vi "TestPrinter.vi"() -> ()   [LabVIEW 2020]
panel:
  in  "ID":string="0"
  in  "SN":string="FFF"
  in  "Print":string
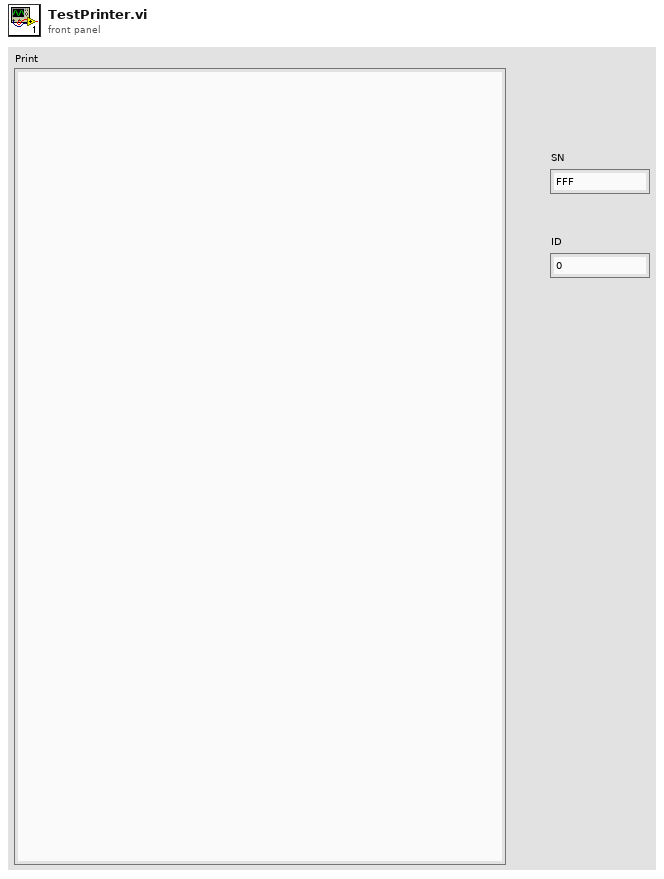
[diagram p1: front panel]
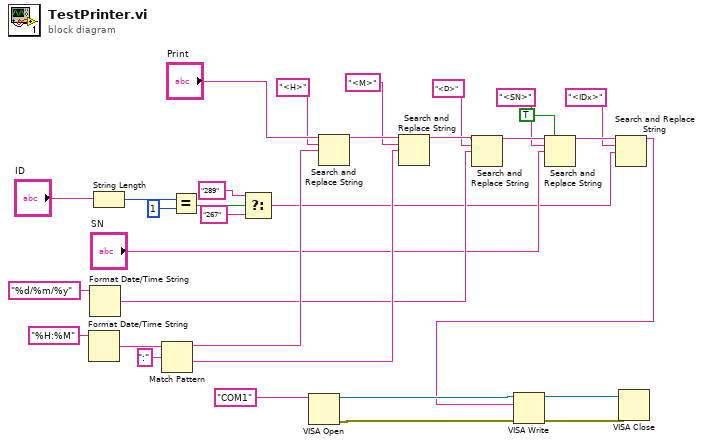
[diagram p0: block diagram]
diagram:
  n1 = Format Date/Time String(time format string (%c)="%H:%M") -> (date/time string=w28:string)  [unwired: 2 in]
  n2 = Format Date/Time String(time format string (%c)="%d/%m/%y") -> (date/time string=w17:string)  [unwired: 2 in]
  n3 = String Length(string="ID") -> (length=w9:i32)
  n4 = Match Pattern(string=w28, regular expression=":") -> (before substring=w22:string, after substring=w19:string)  [unwired: 1 in, 2 out]
  n5 = Equal?(x=w9, y=1) -> (x = y?=w4:bool)
  n6 = Select(t="289", s=w4, f="267") -> (s? t:f=w1:string)
  n7 = VISA Open(VISA resource name="COM1") -> (VISA resource name=w30:refnum<visa-resource-name>, error out=w31:errorcluster)  [unwired: 4 in]
  n8 = Search and Replace String(input string="Print", search string="<H>", replace string=w22) -> (result string=w21:string)  [unwired: 5 in, 3 out]
  n9 = Search and Replace String(input string=w21, search string="<M>", replace string=w19) -> (result string=w16:string)  [unwired: 5 in, 3 out]
  n10 = Search and Replace String(input string=w16, search string="<D>", replace string=w17) -> (result string=w14:string)  [unwired: 5 in, 3 out]
  n11 = Search and Replace String(replace all?=TRUE ("replace all? (F)"), input string=w14, search string="<SN>", replace string="SN") -> (result string=w7:string)  [unwired: 4 in, 3 out]
  n12 = Search and Replace String(input string=w7, search string="<IDx>", replace string=w1) -> (result string=w5:string)  [unwired: 5 in, 3 out]
  n13 = VISA Write(VISA resource name=w30, write buffer=w5, error in (no error)=w31) -> (VISA resource name out=w25:refnum<visa-resource-name>, error out=w26:errorcluster)  [unwired: 1 out]
  n14 = VISA Close(VISA resource name=w25, error in (no error)=w26) -> ()  [unwired: 1 out]
